vi "Excel Get Last Row And Column.vi"(8 "error in (no error)":errorcluster, 11 "report in":refnum<class "NI_report.lvclass">) -> (0 "error out":errorcluster, 1 "Columns":i32, 2 "Rows":i32, 3 "report out":refnum<class "NI_report.lvclass">, 4 "end":cluster{"row":i32, "column":i32})   [LabVIEW 2020, in "varilib.lvlib"]
doc: "Retrieves numbers of rows and columns and the coordinates of the last row and last column in an Excel worksheet."
uses:
  varilib.lvlib
  <vilib>/Utility/NIReport.llb/Excel/NI_Excel.lvclass
  <vilib>/Utility/NIReport.llb/NI_report.lvclass
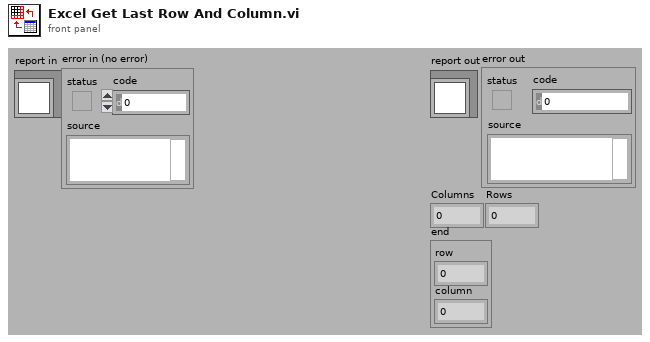
[diagram p1: front panel]
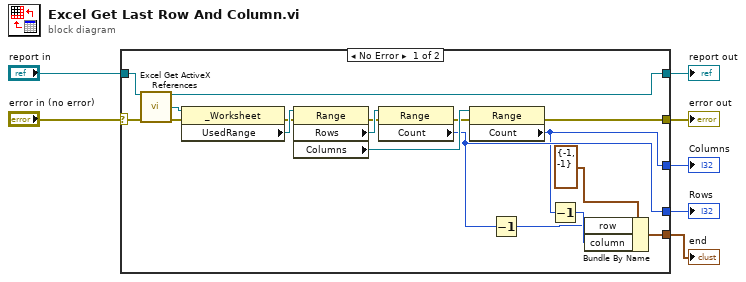
[diagram p0: block diagram]
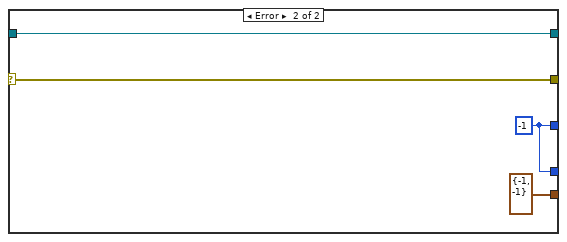
[diagram p2: hidden frame]
diagram:
  n1 = case shown="No Error" "error in (no error)" {
    selector: "error in (no error)" -> [w14 w28]
    tunnel: [w17 w29] -> w7
    tunnel: [w16 w28] -> w6
    tunnel: "report in" -> [w15 w29]
    tunnel: [w8 w27] -> w4
    tunnel: [w9 w27] -> w3
    tunnel: [w10 cluster{"row":i32, "column":i32} {"row"=-1, "column"=-1} ("end (-1, -1)")] -> w1
    frame No Error {
      n2 = call <vilib>:"Excel Get ActiveX References.vi"("report in"=w15, "error in (no error)"=w14) -> ("report out"=w17:refnum<class "NI_report.lvclass">, "Excel._Worksheet"=w19:refnum<k7>, "error out"=w18:errorcluster)  [unwired: 7 in, 4 out]
      n3 = property class="_Worksheet"(reference=w19, error in=w18) -> (error out=w23:errorcluster, "UsedRange"=w24:refnum<k7>)  [unwired: 1 out]
      n4 = property class="Range"(reference=w24, error in=w23) -> (error out=w22:errorcluster, "Rows"=w25:refnum<k7>, "Columns"=w21:refnum<k7>)  [unwired: 1 out]
      n5 = property class="Range"(reference=w25, error in=w22) -> (error out=w20:errorcluster, "Count"=w9:i32)  [unwired: 1 out]
      n6 = property class="Range"(reference=w21, error in=w20) -> (error out=w16:errorcluster, "Count"=w8:i32)  [unwired: 1 out]
      n7 = Decrement(x=w9) -> (x-1=w11:i32)
      n8 = Decrement(x=w8) -> (x-1=w12:i32)
      n9 = Bundle By Name(cluster=cluster{"row":i32, "column":i32} {"row"=-1, "column"=-1} ("end (-1, -1)"), "row"=w11, "column"=w12) -> (w10:cluster{"row":i32, "column":i32})
    }
    frame Error {
      w27 = -1
    }
  }
  "report out" <- w7
  "error out" <- w6
  "Columns" <- w4
  "Rows" <- w3
  "end" <- w1
